vi "Sync Reply.vi"(7 "Sender":refnum<class "Sender.lvclass">, 10 "Msg":refnum<class "Msg.lvclass">, 11 "TEMPLATE Actor in":refnum<class "TEMPLATE Actor.lvclass">) -> (3 "TEMPLATE Actor out":refnum<class "TEMPLATE Actor.lvclass">)   [LabVIEW 2020, in "_Template.lvlib" / "Templates.lvlib" / "TEMPLATE Actor.lvlib" / "TEMPLATE Actor.lvclass"]
uses:
  TEMPLATE Actor.lvclass
  jettl/jettl/Actor/Actor/Actor.lvclass
  jettl/jettl/Sender/Sender/Sender.lvclass
  jettl/jettl/Msg/Msg.lvclass
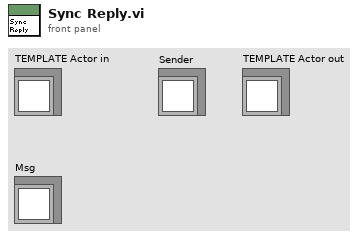
[diagram p1: front panel]
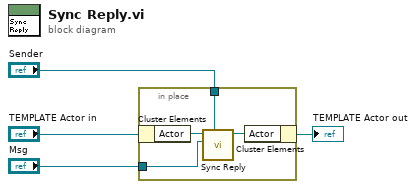
[diagram p0: block diagram]
diagram:
  n1 = in-place {
    in-place-border: "Sender" -> [w6]
    in-place-border: "Msg" -> [w5]
    n2 = in-place-cluster #1("TEMPLATE Actor in") -> ("Actor"=w8:refnum<class "Actor.lvclass">)
    n3 = call-dynamic "Sync Reply.vi"("Sender"=w6, "Msg"=w5, "Actor in"=w8) -> ("Actor out"=w7:refnum<class "Actor.lvclass">)  [unwired: 8 in]
    n4 = in-place-cluster #1("Actor"=w7) -> (→"TEMPLATE Actor out":refnum<class "TEMPLATE Actor.lvclass">)
  }
